vi "SVM.vi"(8 "SVs":i32, 9 "Angle (degrees)":dbl=90.0, 10 "time step":dbl=0.01, 11 "Data IN":dbl[](graph)) -> (0 "A tau":dbl[](array[numeric]), 1 "GapCutOff":i16, 2 "SVM Out":T2 {"eigen lamda" min=0.0 max=127.0 format="%.2e"}, 3 "Array":T1(array[cluster]))   [LabVIEW 2022 SP3]
panel:
  out "Singular Values":dbl[](graph)
  out "Fit to C1":dbl[][](graph)
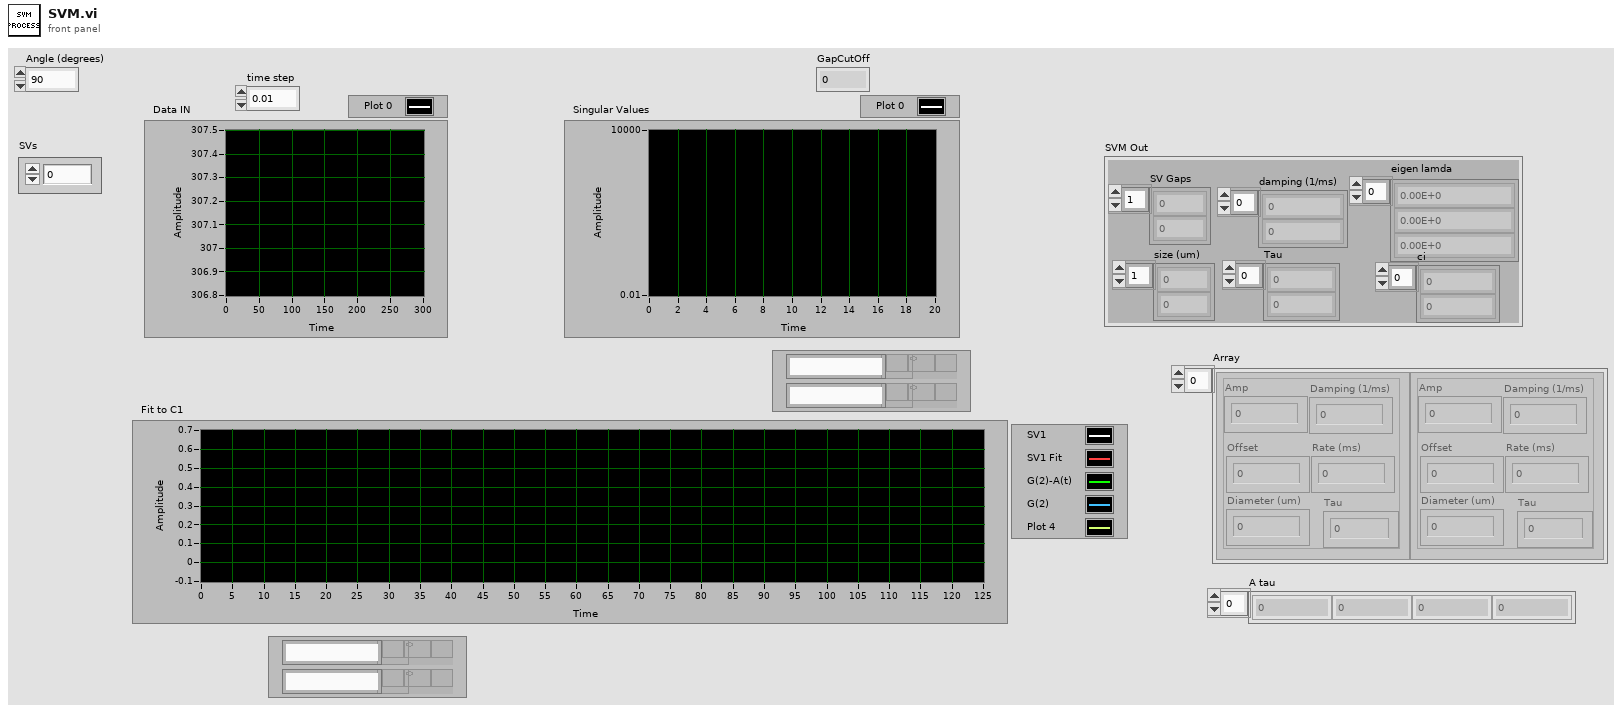
[diagram p1: front panel]
types:
  T1 = cluster{"Amp":dbl, "Offset":dbl, "Damping (1/ms)":dbl, "Rate (ms)":dbl, "Diameter (um)":dbl, "Tau":dbl}[]
  T2 = cluster{"SV Gaps":dbl[], "size (um)":dbl[], "damping (1/ms)":dbl[], "Tau ":cdb[], "eigen lamda":dbl[], "ci":dbl[]}
  T3 = typedef "NI_Matrix.lvlib/RealMatrix.ctl" = dbl[][]
  T4 = cluster{"SV Gap Ratio":dbl[], dbl[], dbl[], cdb[], "eigen lamda":dbl[], "Ci":dbl[]}
  T5 = cluster{"Amp":dbl, "Offset":dbl, "Damping (1/ms)":dbl, "Rate (ms)":dbl, "Diameter (um)":dbl, "Tau":dbl}
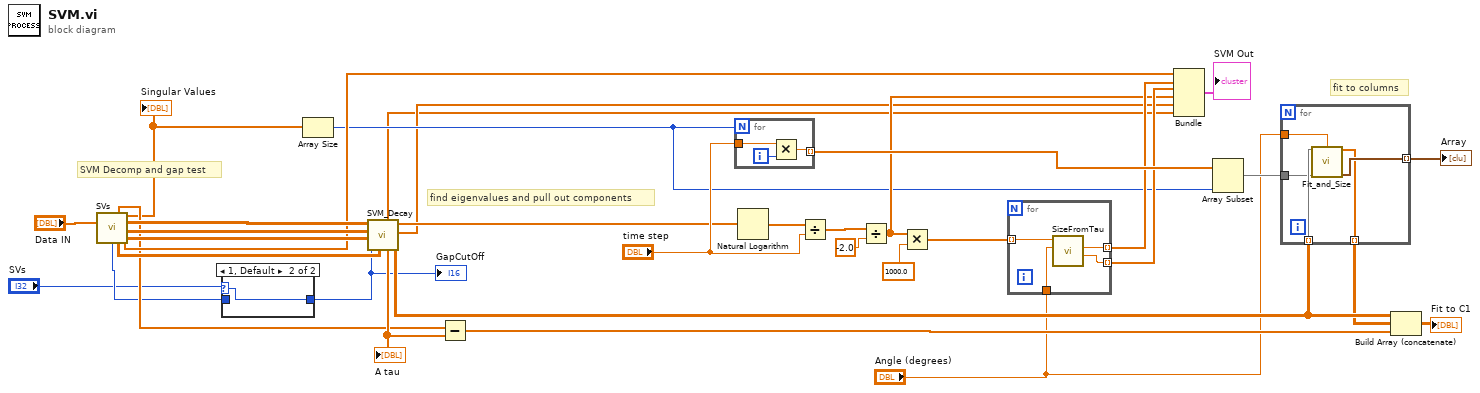
[diagram p0: block diagram]
diagram:
  # "fit to columns"
  # "find eigenvalues and pull out components"
  # "SVM Decomp and gap test"
  n1 = call "SVs.vi"("Data in"="Data IN") -> ("G2"=w13:dbl[], "Singular Values"=w12:dbl[], "Matrix U"=w18:T3, "Matrix S"=w17:T3, "Matrix V"=w16:T3, "GapCutOff"=w3:i16, "Hs"=w15:dbl[][], "SV Gap Ratio"=w14:dbl[])  [unwired: 7 in]
  "Singular Values" <- w12
  n2 = case shown="1, Default" "SVs" {
    selector: "SVs" -> [_ w36]
    tunnel: w3 -> [w35 _]
    tunnel: [w35 w36] -> w2
    frame 0 {
    }
    frame 1, Default {
    }
  }
  "GapCutOff" <- w2
  n3 = Array Size(array=w12) -> (size(s)=w11:i32)
  n4 = call "SVM_Decay.vi"("Hs"=w15, "GapCutOff"=w2, "Matrix V"=w16, "Matrix S"=w17, "Matrix U"=w18) -> ("G2"=w25:dbl[][], "eigen lamda"=w9:dbl[], "Eigenvalues"=w10:cdb[], "A(tau)"=w26:dbl[], "Ci"=w8:dbl[])  [unwired: 2 in]
  "A tau" <- w26
  n5 = Subtract(x=w13, y=w26) -> (x-y=w27:dbl[])
  n6 = for {
    N: w11 -> [_]
    tunnel: [w38] -> w29 mode=indexing
    tunnel: "time step" -> [w37]
    i -> [w39]
    n7 = Multiply(x=w37, y=w39) -> (x*y=w38:dbl)
  }
  n8 = Natural Logarithm ("Natural Logarithm.vi")(1:w10) -> (0:w34:cdb[])
  n9 = Divide(x=w34, y="time step") -> (x/y=w32:cdb[])
  n10 = Divide(x=w32, y=-2.0) -> (x/y=w20:cdb[])
  n11 = Multiply(x=w20, y=1000.0) -> (x*y=w21:cdb[])
  n12 = for {
    tunnel: w21 -> [w43] mode=indexing
    tunnel: [w42] -> w24 mode=indexing
    tunnel: [w41] -> w23 mode=indexing
    tunnel: "Angle (degrees)" -> [w40]
    n13 = call "SizeFromTau.vi"("Angle (degrees)"=w40, "tau 1/s"=w43) -> ("damping (ms)"=w41:dbl, "size (um)"=w42:dbl)  [unwired: 8 in]
  }
  n14 = Bundle("SV Gap Ratio"=w14, w24, w23, w20, "eigen lamda"=w9, "Ci"=w8) -> (→"SVM Out":T4)  [unwired: 1 in]
  n15 = Array Subset(array=w29, length=w11) -> (w7:dbl[])  [unwired: 1 in]
  n16 = for {
    tunnel: w25 -> [w48] mode=indexing
    tunnel: [w47] -> w5 mode=indexing
    tunnel: w7 -> [w46]
    tunnel: [w45] -> w6 mode=indexing
    tunnel: "Angle (degrees)" -> [w44]
    n17 = call "Fit_and_Size.vi"("G2"=w48, "Angle (degrees)"=w44, "Time"=w46) -> ("Best Exponential Fit"=w45:dbl[], "Fit"=w47:T5)  [unwired: 7 in, 4 out]
  }
  "Array" <- w5
  n18 = Build Array (concatenate)(w25, w6, w27) -> (→"Fit to C1":dbl[][])
